vi "HoloPy_get_all_image_files_in_directory.vi"(8 "error in (no error)":errorcluster, 9 "file_extension":string, 10 "holo directory":path, 11 "Refnum in":refnum<k35>) -> (0 "error out":errorcluster, 2 "path":path[](array[path]), 3 "Refnum out":refnum<k35>)   [LabVIEW 2023, in "holoPyTracks.lvlib"]
uses:
  holoPyTracks.lvlib
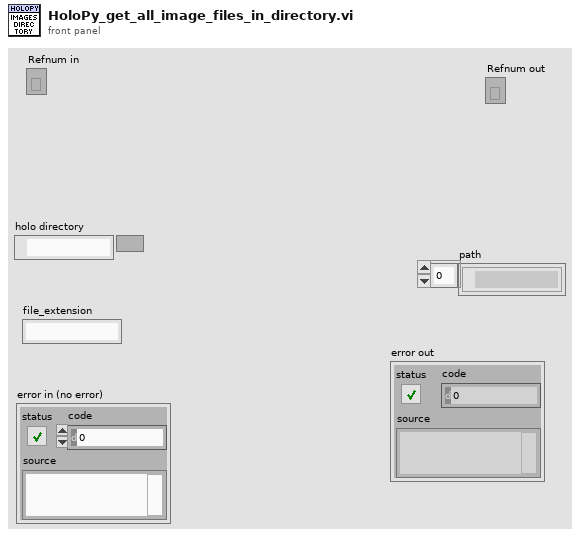
[diagram p1: front panel]
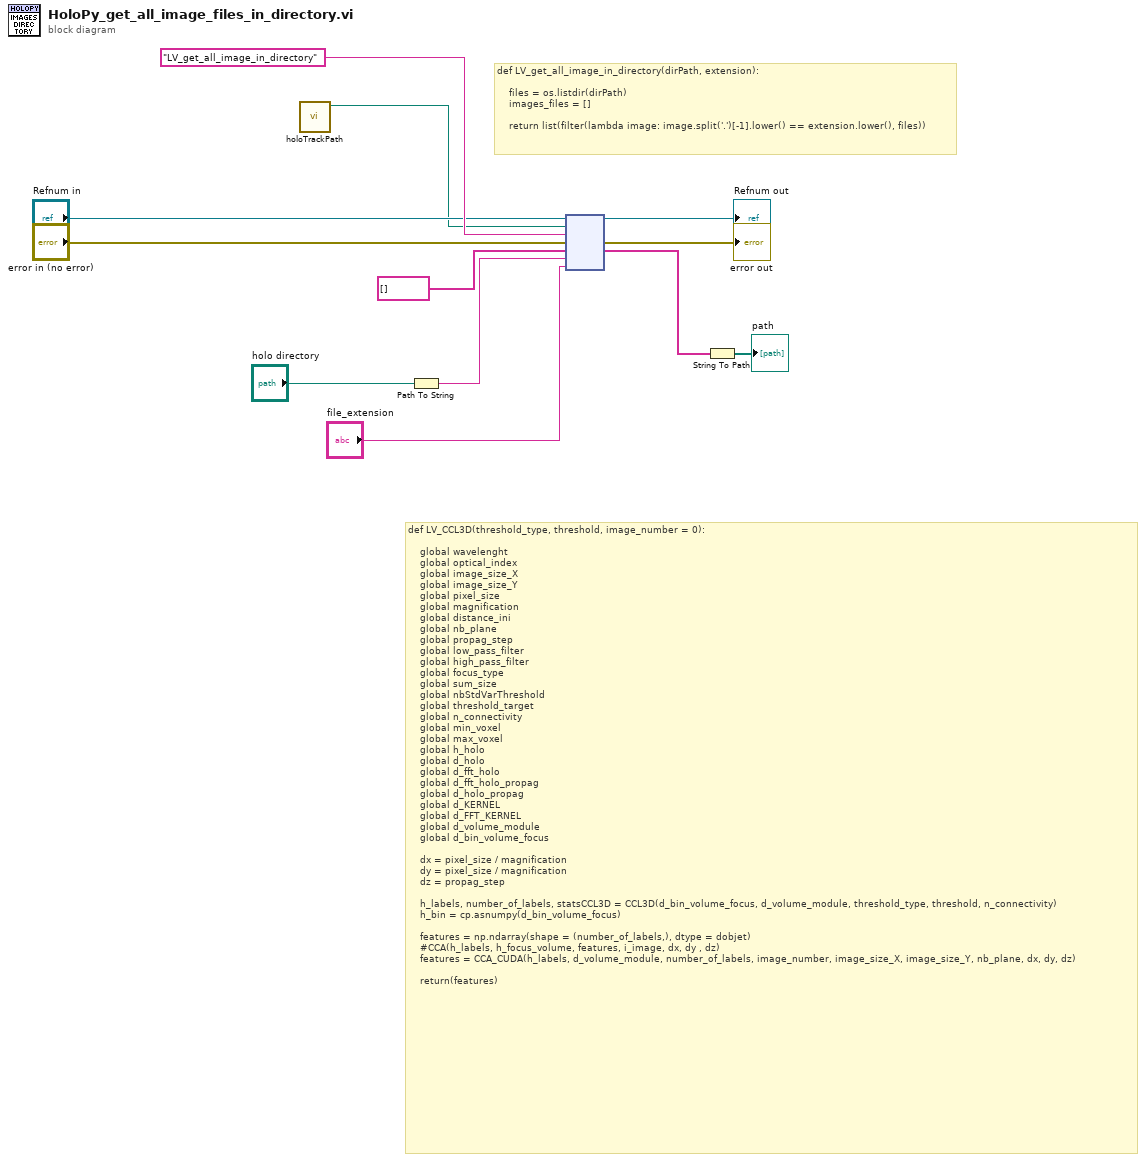
[diagram p0: block diagram]
diagram:
  # "def LV_get_all_image_in_directory(dirPath, extension):\n\n    files = os.listdir(dirPath) \n    images_files = []\n\n    return list(filter(lambda image: image.split('.')[-1].lower() == extension.lower(), files))"
  # "def LV_CCL3D(threshold_type, threshold, image_number = 0):\n\n    global wavelenght \n    global optical_index \n    global image_size_X \n    global image_size_Y \n    global pixel_size \n    global magnification\n    global distance_ini\n    global nb_plane \n    global propag_step \n    global low_pass_filter\n    global high_pass_filter \n    global focus_type\n    global sum_size \n    global nbStdVarThreshold\n    global threshold_target\n    global n_connectivity\n    global min_voxel \n    global max_voxel\n    global h_holo\n    global d_holo\n    global d_fft_holo\n    global d_fft_holo_propag\n    global d_holo_propag\n    global d_KERNEL\n    global d_FFT_KERNEL\n    global d_volume_module\n    global d_bin_volume_focus\n\n    dx = pixel_size / magnification\n    dy = pixel_size / magnification\n    dz = propag_step\n\n    h_labels, number_of_labels, statsCCL3D = CCL3D(d_bin_volume_focus, d_volume_module, threshold_type, threshold, n_connectivity)\n    h_bin = cp.asnumpy(d_bin_volume_focus)\n\n    features = np.ndarray(shape = (number_of_labels,), dtype = dobjet)\n    #CCA(h_labels, h_focus_volume, features, i_image, dx, dy , dz)\n    features = CCA_CUDA(h_labels, d_volume_module, number_of_labels, image_number, image_size_X, image_size_Y, nb_plane, dx, dy, dz)\n\n    return(features)"
  n1 = call "holoTrackPath.vi"() -> ("appended path"=w7:path)  [unwired: 11 in]
  n2 = Path To String(path="holo directory") -> (string=w5:string)
  n3 = node("Refnum in", w7, "LV_get_all_image_in_directory" ("function name"), "error in (no error)", string[] [] ("string"), w5, "file_extension") -> (→"Refnum out":refnum<k35>, →"error out":errorcluster, w3:string[])  [unwired: 2 in, 2 out]
  n4 = String To Path(string=w3) -> (path=→"path":path[])
